vi "Dashboard custom_server communication.vi"() -> ()   [LabVIEW 2017]
uses:
  C:/Users/IMR Lab/Documents/LabVIEW Data/UniversalRobotsSDK_LABView/LabVIEW/Examples/LabVIEW10/UnderAutomation.UniversalRobots.dll
  UnderAutomation.UniversalRobots.dll
panel:
  in  "stop":bool
  in  "TCP switch":bool
  out "Rx":dbl
  out "Rz":dbl
  out "Ry":dbl
  out "Enabled":bool
  out "Port":i32
  in  "Move to particular posture":bool
  in  "Move to Zero position":bool
  out "Connected":bool
  in  "Robot IP(192.168.112.182)":string
  out "Connect error":errorcluster
  in  "Power on\nRelease brake":bool
  in  "Power off":bool
  in  "Connect":bool
  in  "Send script":bool
  in  "Script to execute":string
  out "Powered on":bool
  out "X":dbl
  out "Y":dbl
  out "Z":dbl
  out "License state":string
  # "movel(p[-0.0753945, -0.304532, 0.314608, -0.194623, 2.71667, -1.00228], a= 0.5, v=0.25)"
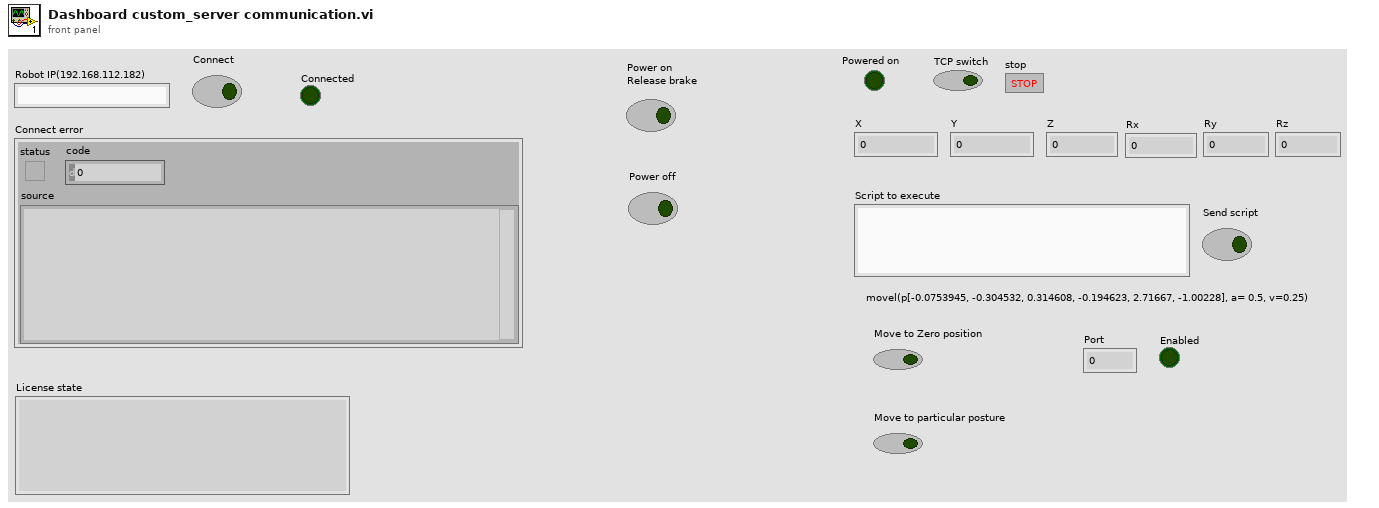
[diagram p1: front panel]
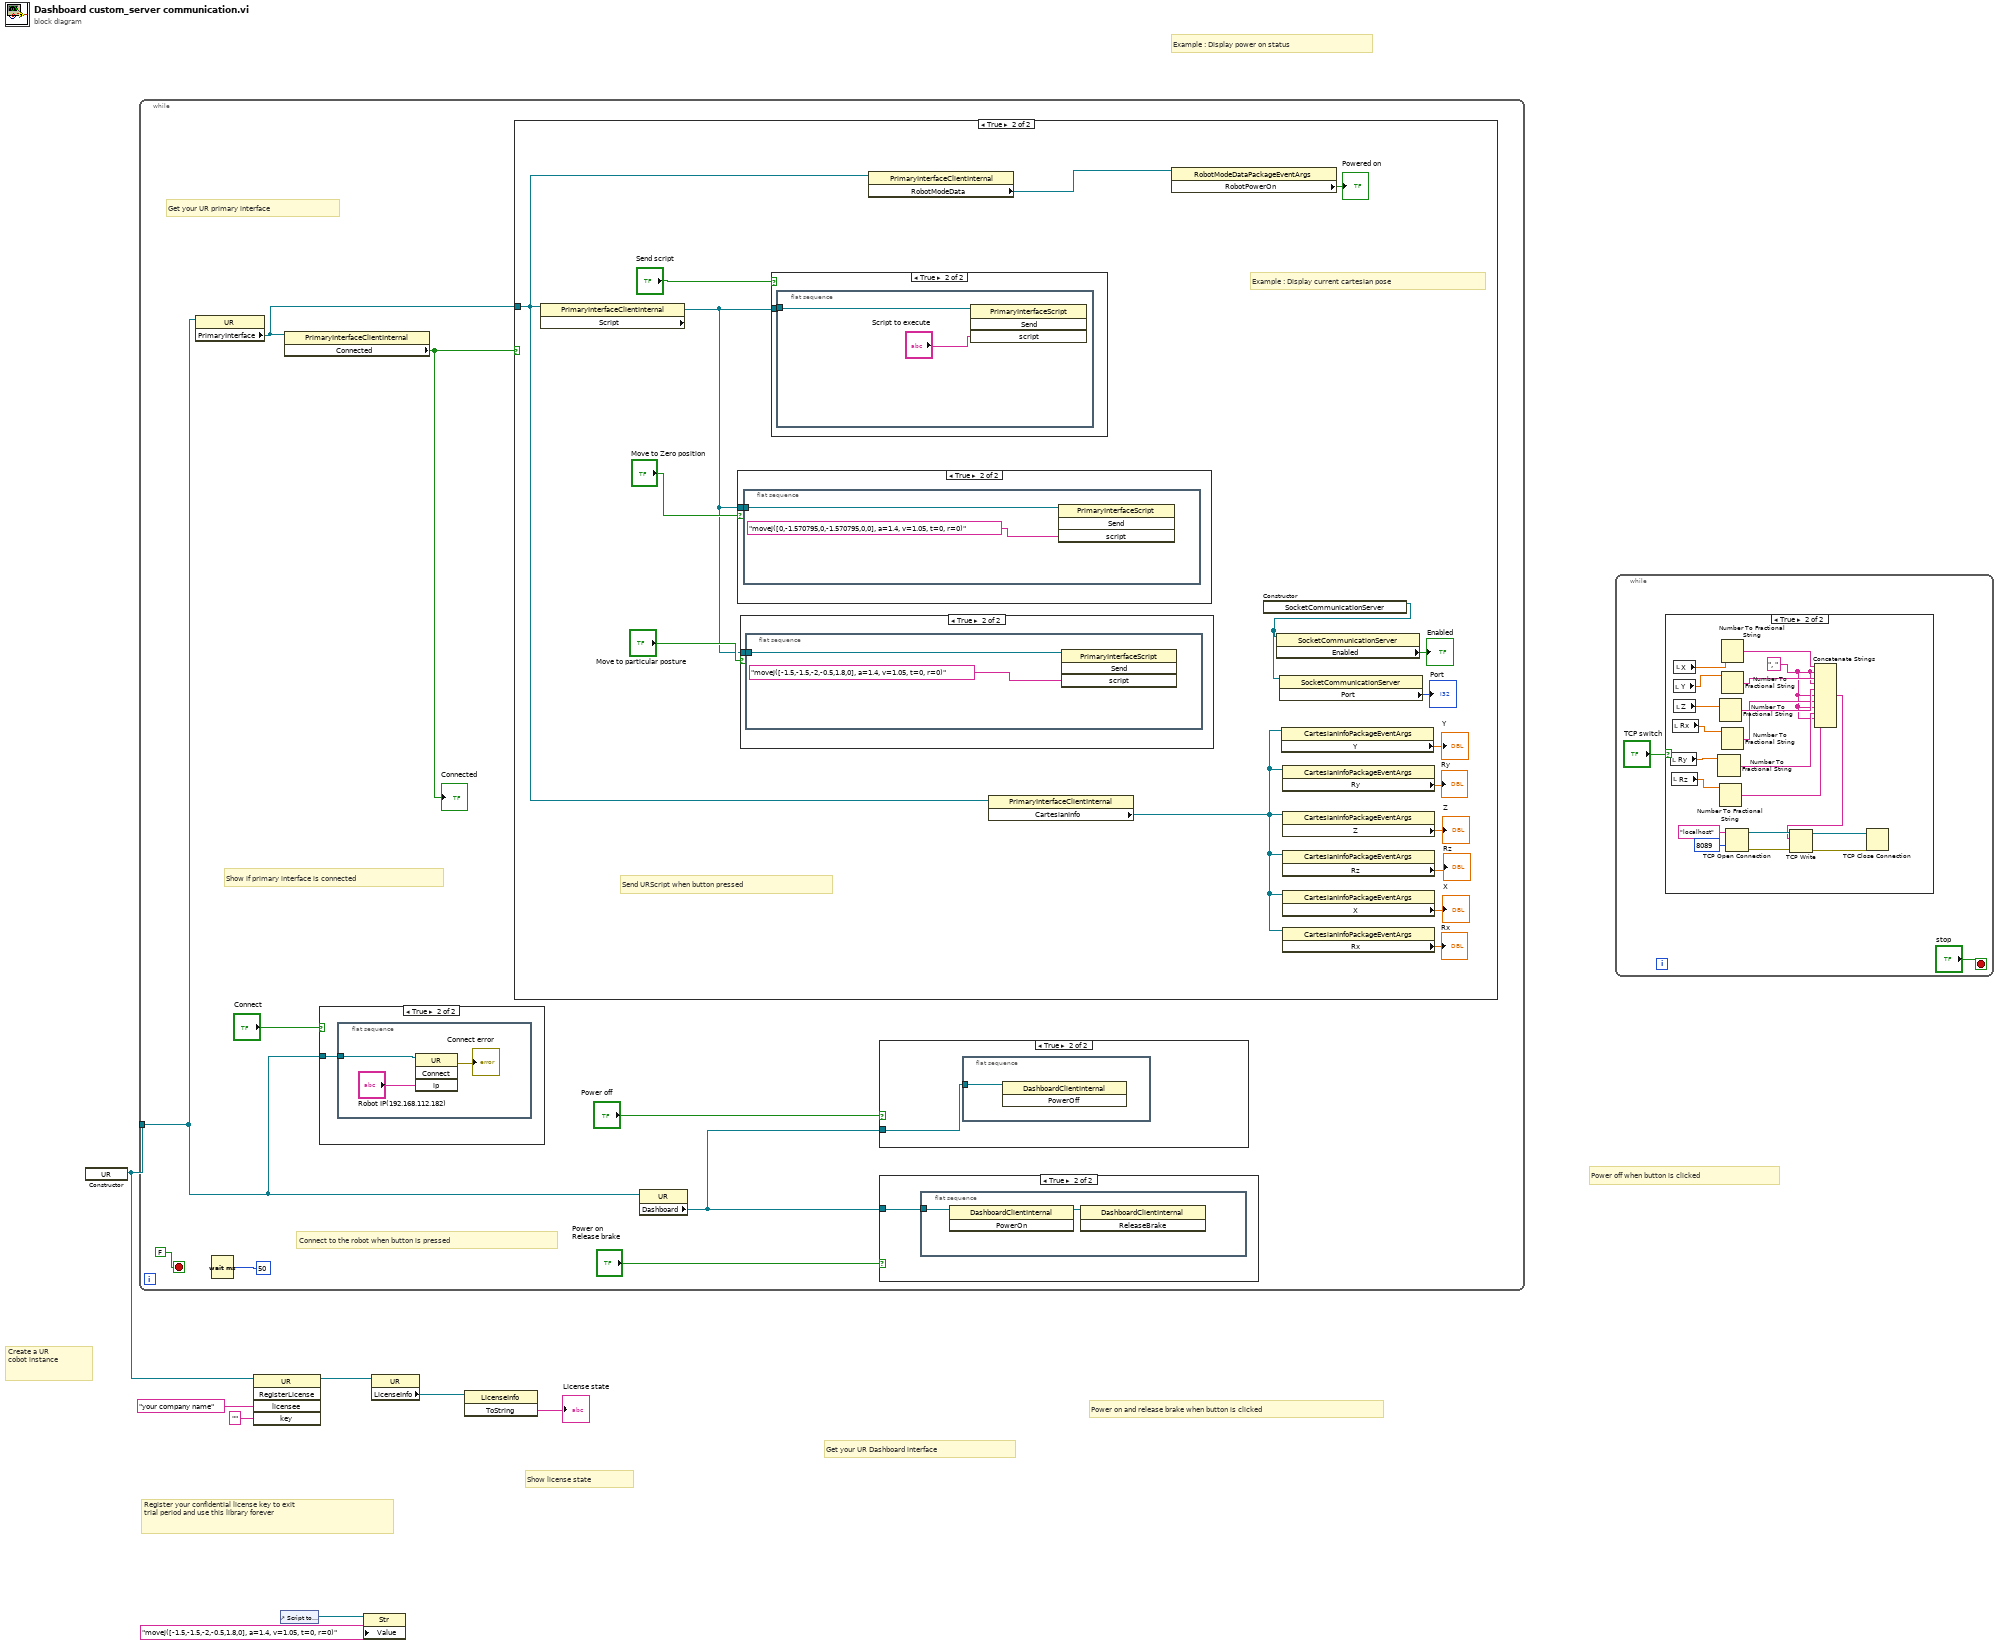
[diagram p0: block diagram]
diagram:
  # "Example : Display power on status"
  # "Create a UR\ncobot instance"
  # "Show license state"
  # "Register your confidential license key to exit\ntrial period and use this library forever"
  # "Power off when button is clicked"
  # "Power on and release brake when button is clicked"
  # "Get your UR Dashboard interface"
  n1 = constructor class="UR"() -> (reference out=w3:refnum<k24>)  [unwired: 3 in, 2 out]
  n2 = while {
    tunnel: w3 -> [w9]
    stop <- FALSE stop-if-true
    # "Connect to the robot when button is pressed"
    # "Show if primary interface is connected"
    # "Get your UR primary interface"
    n3 = property class="UR"(reference=w9) -> ("PrimaryInterface"=w12:refnum<k24>)  [unwired: 1 in, 2 out]
    n4 = Wait (ms)(milliseconds to wait=u32 50) -> ()  [unwired: 1 out]
    n5 = property class="PrimaryInterfaceClientInternal"(reference=w12) -> ("Connected"=w11:bool)  [unwired: 1 in, 2 out]
    "Connected" <- w11
    n6 = case shown="True" "Connect" {
      tunnel: w9 -> [_ w49]
      frame False {
      }
      frame True {
        n7 = flat-sequence {
          tunnel: w49 -> [w51]
          frame #0 {
            n8 = invoke class="UR" method="Connect"(reference=w51, "ip"="Robot IP(192.168.112.182)") -> (error out=→"Connect error":errorcluster)  [unwired: 2 in, 3 out]
          }
        }
      }
    }
    n9 = case shown="True" w11 {
      tunnel: w12 -> [_ w28]
      frame False {
      }
      frame True {
        # "Send URScript when button pressed"
        # "Example : Display current cartesian pose"
        n10 = property class="PrimaryInterfaceClientInternal"(reference=w28) -> ("Script"=w25:refnum<k24>)  [unwired: 1 in, 2 out]
        n11 = case shown="True" "Move to Zero position" {
          tunnel: w25 -> [_ w38]
          frame False {
          }
          frame True {
            n12 = flat-sequence {
              tunnel: w38 -> [w40]
              frame #0 {
                n13 = invoke class="PrimaryInterfaceScript" method="Send"(reference=w40, "script"="movej([0,-1.570795,0,-1.570795,0,0], a=1.4, v=1.05, t=0, r=0)") -> ()  [unwired: 2 in, 4 out]
              }
            }
          }
        }
        n14 = case shown="True" "Move to particular posture" {
          tunnel: w25 -> [_ w35]
          frame False {
          }
          frame True {
            n15 = flat-sequence {
              tunnel: w35 -> [w37]
              frame #0 {
                n16 = invoke class="PrimaryInterfaceScript" method="Send"(reference=w37, "script"="movej([-1.5,-1.5,-2,-0.5,1.8,0], a=1.4, v=1.05, t=0, r=0)") -> ()  [unwired: 2 in, 4 out]
              }
            }
          }
        }
        n17 = case shown="True" "Send script" {
          tunnel: w25 -> [_ w41]
          frame False {
          }
          frame True {
            n18 = flat-sequence {
              tunnel: w41 -> [w43]
              frame #0 {
                n19 = invoke class="PrimaryInterfaceScript" method="Send"(reference=w43, "script"="Script to execute") -> ()  [unwired: 2 in, 4 out]
              }
            }
          }
        }
        n20 = property class="PrimaryInterfaceClientInternal"(reference=w28) -> ("RobotModeData"=w33:refnum<k24>)  [unwired: 1 in, 2 out]
        n21 = property class="PrimaryInterfaceClientInternal"(reference=w28) -> ("CartesianInfo"=w19:refnum<k24>)  [unwired: 1 in, 2 out]
        n22 = property class="RobotModeDataPackageEventArgs"(reference=w33) -> ("RobotPowerOn"=→"Powered on":bool)  [unwired: 1 in, 2 out]
        n23 = constructor class="SocketCommunicationServer"() -> (reference out=w24:refnum<k24>)  [unwired: 3 in, 2 out]
        n24 = property class="SocketCommunicationServer"(reference=w24) -> ("Enabled"=→"Enabled":bool)  [unwired: 1 in, 2 out]
        n25 = property class="SocketCommunicationServer"(reference=w24) -> ("Port"=→"Port":i32)  [unwired: 1 in, 2 out]
        n26 = property class="CartesianInfoPackageEventArgs"(reference=w19) -> ("Y"=→"Y":dbl)  [unwired: 1 in, 2 out]
        n27 = property class="CartesianInfoPackageEventArgs"(reference=w19) -> ("Ry"=→"Ry":dbl)  [unwired: 1 in, 2 out]
        n28 = property class="CartesianInfoPackageEventArgs"(reference=w19) -> ("Z"=→"Z":dbl)  [unwired: 1 in, 2 out]
        n29 = property class="CartesianInfoPackageEventArgs"(reference=w19) -> ("Rz"=→"Rz":dbl)  [unwired: 1 in, 2 out]
        n30 = property class="CartesianInfoPackageEventArgs"(reference=w19) -> ("X"=→"X":dbl)  [unwired: 1 in, 2 out]
        n31 = property class="CartesianInfoPackageEventArgs"(reference=w19) -> ("Rx"=→"Rx":dbl)  [unwired: 1 in, 2 out]
      }
    }
    n32 = property class="UR"(reference=w9) -> ("Dashboard"=w13:refnum<k24>)  [unwired: 1 in, 2 out]
    n33 = case shown="True" "Power off" {
      tunnel: w13 -> [_ w44]
      frame False {
      }
      frame True {
        n34 = flat-sequence {
          tunnel: w44 -> [w45]
          frame #0 {
            n35 = invoke class="DashboardClientInternal" method="PowerOff"(reference=w45) -> ()  [unwired: 2 in, 3 out]
          }
        }
      }
    }
    n36 = case shown="True" "Power on\nRelease brake" {
      tunnel: w13 -> [_ w46]
      frame False {
      }
      frame True {
        n37 = flat-sequence {
          tunnel: w46 -> [w48]
          frame #0 {
            n38 = invoke class="DashboardClientInternal" method="PowerOn"(reference=w48) -> (reference out=w47:refnum<k24>)  [unwired: 2 in, 2 out]
            n39 = invoke class="DashboardClientInternal" method="ReleaseBrake"(reference=w47) -> ()  [unwired: 2 in, 3 out]
          }
        }
      }
    }
  }
  n40 = invoke class="UR" method="RegisterLicense"(reference=w3, "licensee"="your company name", "key"="") -> (reference out=w5:refnum<k24>)  [unwired: 2 in, 4 out]
  n41 = control-ref of="Script to execute"() -> (w2:refnum<vi>)
  n42 = property class="Str"(reference=w2, "Value"="movej([-1.5,-1.5,-2,-0.5,1.8,0], a=1.4, v=1.05, t=0, r=0)") -> ()  [unwired: 1 in, 2 out]
  n43 = property class="UR"(reference=w5) -> ("LicenseInfo"=w4:refnum<k24>)  [unwired: 1 in, 2 out]
  n44 = invoke class="LicenseInfo" method="ToString"(reference=w4) -> ("ToString"=→"License state":string)  [unwired: 2 in, 2 out]
  n45 = while {
    stop <- "stop" stop-if-true
    n46 = case shown="True" "TCP switch" {
      frame False {
      }
      frame True {
        w57 = ", "
        n47 = local read "Ry"() -> (w64:dbl)
        n48 = local read "Rz"() -> (w63:dbl)
        n49 = local read "Rx"() -> (w65:dbl)
        n50 = local read "Y"() -> (w67:dbl)
        n51 = local read "X"() -> (w68:dbl)
        n52 = local read "Z"() -> (w66:dbl)
        n53 = Number To Fractional String(number=w64) -> (F-format string=w58:string)  [unwired: 3 in]
        n54 = Number To Fractional String(number=w66) -> (F-format string=w60:string)  [unwired: 3 in]
        n55 = Number To Fractional String(number=w63) -> (F-format string=w56:string)  [unwired: 3 in]
        n56 = Number To Fractional String(number=w68) -> (F-format string=w62:string)  [unwired: 3 in]
        n57 = Number To Fractional String(number=w67) -> (F-format string=w61:string)  [unwired: 3 in]
        n58 = Number To Fractional String(number=w65) -> (F-format string=w59:string)  [unwired: 3 in]
        n59 = TCP Open Connection(address="localhost", remote port or service name=u16 8089) -> (connection ID=w72:refnum<k5>, error out=w71:errorcluster)  [unwired: 3 in]
        n60 = Concatenate Strings(w62, w57, w61, w57, w60, w57, w59, w57, w58, w57, w56) -> (w55:string)
        n61 = TCP Write(connection ID=w72, data in=w55, error in (no error)=w71) -> (connection ID out=w70:refnum<k5>, error out=w69:errorcluster)  [unwired: 1 in, 1 out]
        n62 = TCP Close Connection(connection ID=w70, error in (no error)=w69) -> ()  [unwired: 1 in, 2 out]
      }
    }
  }
